vi "EX7-2_DC motor control_PWM.vi"() -> ()   [LabVIEW 2011]
uses:
  <vilib>/LabVIEW Interface for Arduino/LabVIEW Interface for Arduino.lvlib
panel:
  in  "Speed":u32(knob) scale=0.0..255.0
  out "Ready?":bool
  in  "stop":bool
  in  "Selection":T1(radio)
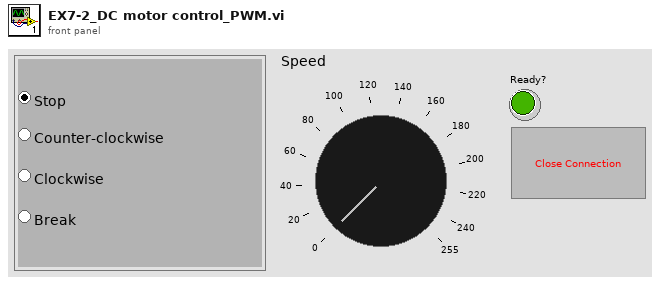
[diagram p1: front panel]
types:
  T1 = enum32{"Stop", "Clockwise", "Counter-clockwise", "Break"}
  T2 = typedef "LabVIEW Interface for Arduino.lvlib/Arduino Resource.ctl" = cluster{"VISA resource":refnum<visa-resource-name>, "Board Type":T3, "Connection Type":enum8{"USB / Serial"}, "Bytes Per Packet (15)":u8}
  T3 = typedef "LabVIEW Interface for Arduino.lvlib/Board Type.ctl" = enum16{"Uno", "Dimuelanove w/Atmega 328", "Mega 2560"}
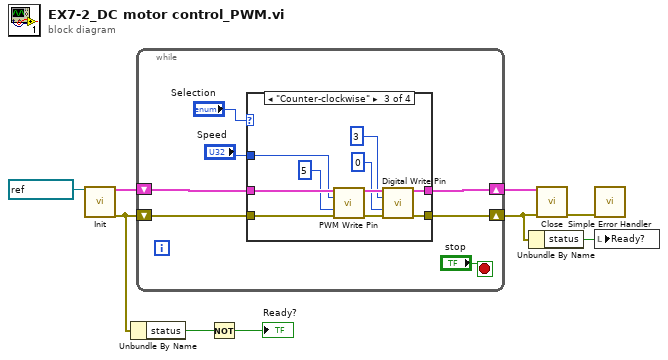
[diagram p0: block diagram]
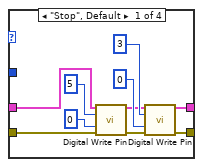
[diagram p2: hidden frame]
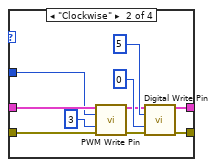
[diagram p3: hidden frame]
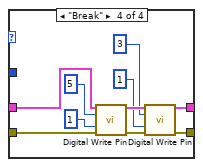
[diagram p4: hidden frame]
diagram:
  n1 = call <vilib>:"Init.vi"("VISA resource"=refnum<visa-resource-name> "COM9") -> ("Arduino Resource"=w8:T2, "error out"=w3:errorcluster)  [unwired: 17 in]
  n2 = Unbundle By Name(w3) -> ("status"=w4:bool)
  n3 = while {
    shift-right: [w13] -> w7
    shift-left: w8 -> [w15]
    shift-right: [w12] -> w2
    shift-left: w3 -> [w14]
    stop <- "stop" stop-if-true
    n4 = case shown="\"Counter-clockwise\"" "Selection" {
      tunnel: w15 -> [w21 w33 w42 w50]
      tunnel: w14 -> [w20 w31 w41 w49]
      tunnel: [w19 w29 w40 w48] -> w13
      tunnel: [w18 w27 w39 w47] -> w12
      tunnel: "Speed" -> [_ w32 w37 _]
      frame "Stop", Default {
        n5 = call <vilib>:"Digital Write Pin.vi"("Arduino Resource"=w21, "Digital I/O Pin (0)"=u8 5, "Value (0)"=u8 0, "error in"=w20) -> ("Arduino Resource"=w17:T2, "error out"=w26:errorcluster)  [unwired: 10 in]
        n6 = call <vilib>:"Digital Write Pin.vi"("Arduino Resource"=w17, "Digital I/O Pin (0)"=u8 3, "Value (0)"=u8 0, "error in"=w26) -> ("Arduino Resource"=w19:T2, "error out"=w18:errorcluster)  [unwired: 10 in]
      }
      frame "Clockwise" {
        n7 = call <vilib>:"PWM Write Pin.vi"("Arduino Resource"=w33, "Duty Cycle (0 - 255)"=w32, "PWM Pin (3)"=u8 3 ("Digital I/O Pin (0)"), "error in"=w31) -> ("Arduino Resource"=w30:T2, "error out"=w28:errorcluster)  [unwired: 10 in]
        n8 = call <vilib>:"Digital Write Pin.vi"("Arduino Resource"=w30, "Digital I/O Pin (0)"=u8 5, "Value (0)"=u8 0, "error in"=w28) -> ("Arduino Resource"=w29:T2, "error out"=w27:errorcluster)  [unwired: 10 in]
      }
      frame "Counter-clockwise" {
        n9 = call <vilib>:"PWM Write Pin.vi"("Arduino Resource"=w42, "Duty Cycle (0 - 255)"=w37, "PWM Pin (3)"=u8 5 ("Digital I/O Pin (0)"), "error in"=w41) -> ("Arduino Resource"=w45:T2, "error out"=w46:errorcluster)  [unwired: 10 in]
        n10 = call <vilib>:"Digital Write Pin.vi"("Arduino Resource"=w45, "Digital I/O Pin (0)"=u8 3, "Value (0)"=u8 0, "error in"=w46) -> ("Arduino Resource"=w40:T2, "error out"=w39:errorcluster)  [unwired: 10 in]
      }
      frame "Break" {
        n11 = call <vilib>:"Digital Write Pin.vi"("Arduino Resource"=w50, "Digital I/O Pin (0)"=u8 5, "Value (0)"=u8 1, "error in"=w49) -> ("Arduino Resource"=w55:T2, "error out"=w56:errorcluster)  [unwired: 10 in]
        n12 = call <vilib>:"Digital Write Pin.vi"("Arduino Resource"=w55, "Digital I/O Pin (0)"=u8 3, "Value (0)"=u8 1, "error in"=w56) -> ("Arduino Resource"=w48:T2, "error out"=w47:errorcluster)  [unwired: 10 in]
      }
    }
  }
  n13 = Not(x=w4) -> (.not. x?=→"Ready?":bool)
  n14 = Unbundle By Name(w2) -> ("status"=w1:bool)
  n15 = call <vilib>:"Close.vi"("Arduino Resource"=w7, "error in"=w2) -> ("error out"=w6:errorcluster)  [unwired: 13 in]
  n16 = call <vilib>:"Simple Error Handler.vi"("error in (no error)"=w6) -> ()  [unwired: 4 in, 5 out]
  n17 = local write "Ready?"(w1) -> ()
